vi "Compass (SubVI).vi"(1 "Gyro Angle":dbl) -> (0 "Compass Angle":dbl)   [LabVIEW 2014]
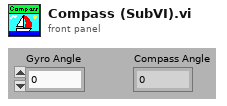
[diagram p1: front panel]
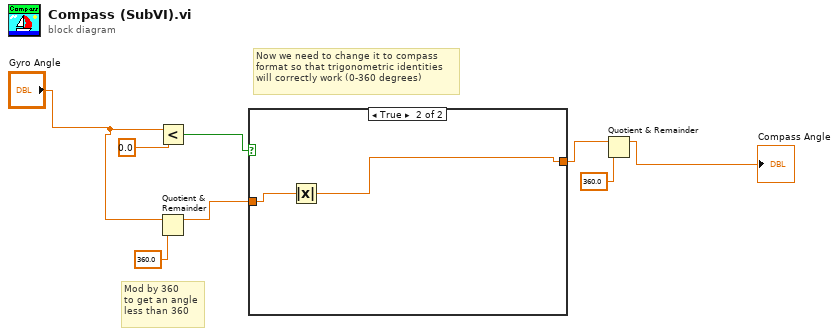
[diagram p0: block diagram]
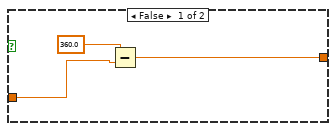
[diagram p2: hidden frame]
diagram:
  # "Mod by 360\nto get an angle\nless than 360"
  # "Now we need to change it to compass\nformat so that trigonometric identities\nwill correctly work (0-360 degrees)"
  n1 = Less?(x="Gyro Angle", y=0.0) -> (x < y?=w5:bool)
  n2 = Quotient & Remainder(x="Gyro Angle", y=360.0) -> (x-y*floor(x/y)=w7:dbl)  [unwired: 1 out]
  n3 = case shown="True" w5 {
    tunnel: [w10 w12] -> w2
    tunnel: w7 -> [w9 w13]
    frame False {
      n4 = Subtract(x=360.0, y=w9) -> (x-y=w10:dbl)
    }
    frame True {
      n5 = Absolute Value(x=w13) -> (abs(x)=w12:dbl)
    }
  }
  n6 = Quotient & Remainder(x=w2, y=360.0) -> (x-y*floor(x/y)=→"Compass Angle":dbl)  [unwired: 1 out]
